vi "StopRequest.vi"(8 "error in (no error)":errorcluster, 9 "Wait for Module to stop? (F)":bool, 11 "ModuleAdmin":refnum<class "ModuleAdmin.lvclass">) -> (0 "error out":errorcluster, 2 "Stop Request Sent":bool)   [LabVIEW 2018, in "ScopeModule.lvlib"]
uses:
  ScopeModule.lvlib
  <userlib>/NIST/ModuleAdminLib/ModuleAdmin/ModuleAdmin.lvclass
  <vilib>/event_ctls.llb/usereventprio.ctl
  PublicAPI/Arguments/Requests/clStopArgument.ctl
  clEventType.ctl
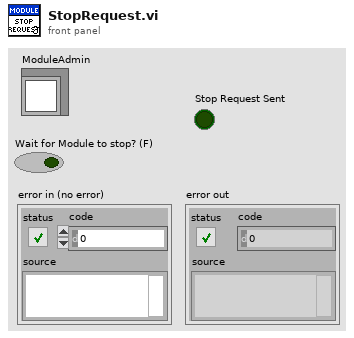
[diagram p1: front panel]
types:
  T1 = typedef "ScopeModule.lvlib/clRequestEvents.ctl" = cluster{"StopRequest":refnum<user-event>, "PathToINI":refnum<user-event>, " LoadPlugin":refnum<user-event>, "ShowPanel":refnum<user-event>, "Abort":refnum<user-event>, "SetAcquisition":refnum<user-event>, "SetChannel":refnum<user-event>, "SetTrigger":refnum<user-event>, "GetAcquisition":refnum<user-event>, "GetChannel":refnum<user-event>, "GetTrigger":refnum<user-event>, "FetchWaveform":refnum<user-event>, "InitAcquisition":refnum<user-event>, "ReadWaveform":refnum<user-event>, "GetHandle":refnum<user-event>, "SetHandle":refnum<user-event>, "GetModel":refnum<user-event>, "SetModel":refnum<user-event>, "ConfigAquisition":refnum<user-event>, "ConfigChannels":refnum<user-event>, "ConfigTrigger":refnum<user-event>, "Initialize":refnum<user-event>, "SetExtAcquisition":refnum<user-event>, "StopAcquisition":refnum<user-event>, "PrefDlg":refnum<user-event>, "Close":refnum<user-event>, "SetSync":refnum<user-event>}
  T2 = typedef "ScopeModule.lvlib/clEventType.ctl" = cluster{"ModuleID":i32, "Data":variant}
  T3 = typedef "ScopeModule.lvlib/clStopArgument.ctl" = cluster{"Exit via Stop Module Req?":bool, "Wait for Module to stop?":bool, "ModuleAdmin":refnum<class "ModuleAdmin.lvclass">}
  T4 = typedef "usereventprio.ctl" = enum32{"high priority", "normal priority"}
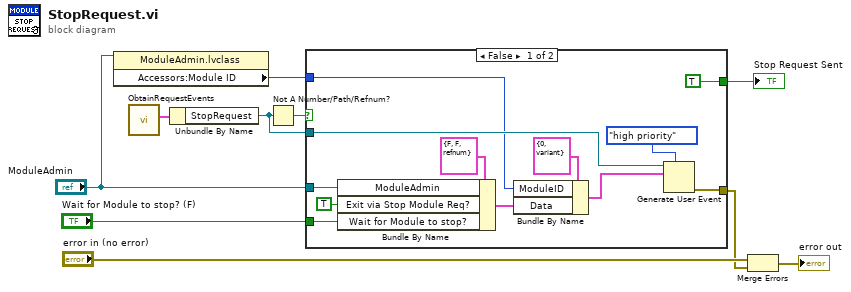
[diagram p0: block diagram]
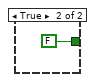
[diagram p2: hidden frame]
diagram:
  n1 = property class="ModuleAdmin.lvclass"(reference="ModuleAdmin") -> ("Accessors:Module ID"=w2:i32)  [unwired: 1 in, 2 out]
  n2 = call "ObtainRequestEvents.vi"() -> ("ScopeRequests"=w10:T1)  [unwired: 10 in, 1 out]
  n3 = Unbundle By Name(w10) -> ("StopRequest"=w8:refnum<user-event>)
  n4 = Not A Number/Path/Refnum?(number/path/refnum=w8) -> (NaN/Path/Refnum?=w9:bool)
  n5 = case shown="False" w9 {
    tunnel: w8 -> [w22 _]
    tunnel: "ModuleAdmin" -> [w15 _]
    tunnel: "Wait for Module to stop? (F)" -> [w14 _]
    tunnel: [w13 _] -> w4
    tunnel: w2 -> [w12 _]
    tunnel: [TRUE FALSE] -> w1
    frame False {
      n6 = Bundle By Name(cluster=T3 {"Exit via Stop Module Req?"=FALSE, "Wait for Module to stop?"=FALSE, "ModuleAdmin"=refnum} ("Stop Argument"), "ModuleAdmin"=w15, "Exit via Stop Module Req?"=TRUE, "Wait for Module to stop?"=w14) -> (w17:T3)
      n7 = Bundle By Name(cluster=T2 {"ModuleID"=0, "Data"=variant} ("clBroadcast"), "ModuleID"=w12, "Data"=w17) -> (w16:T2)
      n8 = Generate User Event(priority (normal)=usereventprio."high priority", user event=w22, event data cluster=w16) -> (error out=w13:errorcluster)  [unwired: 1 in, 1 out]
    }
    frame True {
    }
  }
  "Stop Request Sent" <- w1
  n9 = Merge Errors("error in (no error)", w4) -> (→"error out":errorcluster)
